vi "Emballage_BDD_choix_Config_GVF_ref.vi"(8 "Error in":errorcluster caption="Error in (no error)", 10 "Énum":enum16{"get", "set"}(ring), 11 "Cluster IN":T1) -> (0 "Error out":errorcluster, 3 "Cluster OUT":T1)   [LabVIEW 2020]
uses:
  Choix_Config_ref.ctl
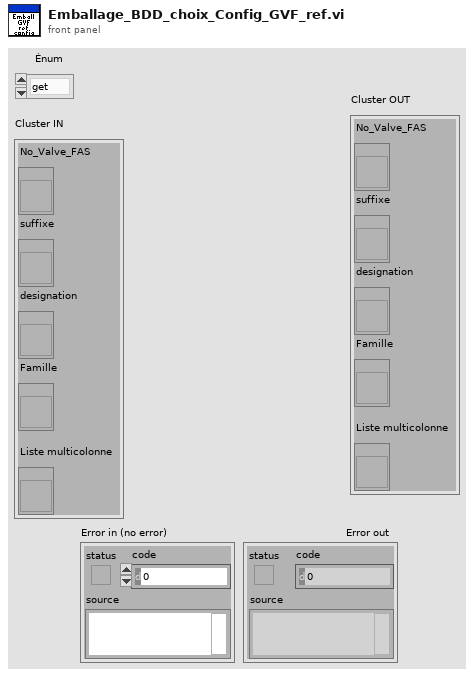
[diagram p1: front panel]
types:
  T1 = typedef "Choix_Config_ref.ctl" = cluster{"No_Valve_FAS":refnum<vi>, "Liste multicolonne":refnum<vi>, "suffixe":refnum<vi>, "designation":refnum<vi>, "Famille":refnum<vi>}
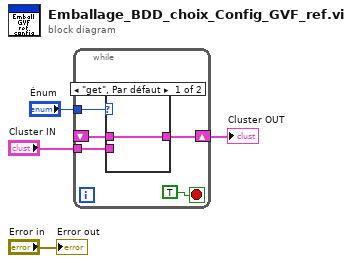
[diagram p0: block diagram]
diagram:
  n1 = while {
    tunnel: "Énum" -> [w8]
    tunnel: "Cluster IN" -> [w6]
    shift-right: [w7] -> w1
    shift-left: _ -> [w5]
    stop <- TRUE stop-if-true
    n2 = case shown="\"get\", Par défaut" w8 {
      tunnel: [w10 w11] -> w7
      tunnel: w6 -> [_ w11]
      tunnel: w5 -> [w10 _]
      frame "get", Default {
      }
      frame "set" {
      }
    }
  }
  "Cluster OUT" <- w1
  "Error out" <- "Error in"
